vi "drive_get_distance.vi"(9 "Wheel Radius":dbl, 10 "Reset?":bool, 11 "Current Rotations":dbl) -> (3 "Actual Distance":dbl)   [LabVIEW 2013]
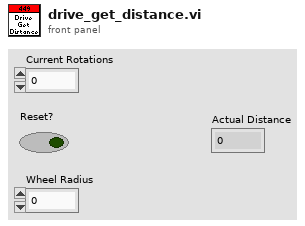
[diagram p1: front panel]
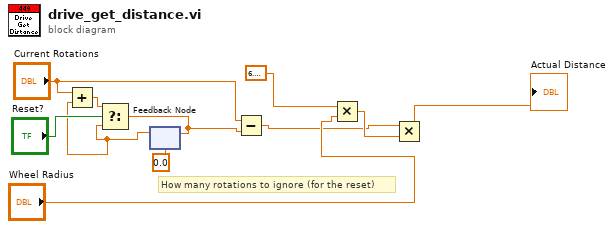
[diagram p0: block diagram]
diagram:
  # "How many rotations to ignore (for the reset)"
  n1 = feedback #1(0.0) -> (w6:dbl)
  n2 = Add(x="Current Rotations", y=w6) -> (x+y=w7:dbl)
  n3 = Select(t=w7, s="Reset?", f=w6) -> (s? t:f=w3:dbl)
  n4 = feedback-in #1(w3) -> ()
  n5 = Subtract(x="Current Rotations", y=w3) -> (x-y=w1:dbl)
  n6 = Multiply(x=6.283185307179586, y="Wheel Radius") -> (x*y=w10:dbl)
  n7 = Multiply(x=w1, y=w10) -> (x*y=→"Actual Distance":dbl)
